vi "SSL Detection Frame Simple Estimator Kalman.vi"(7 "Enable":bool, 10 "Field Size":T1, 11 "Detection Frame In":T2 {"robots_blue"."height" format="%+4.3f"; "robots_blue"."pixel_y" format="%+4.3f"; "robots_blue"."pixel_x" format="%+4.3f"; "robots_blue"."orientation" format="%+4.3f"; "robots_blue"."y" format="%+4.3f"; "robots_blue"."confidence" format="%4.3f"; "robots_blue"."x" format="%+4.3f"; "robots_yellow"."height" format="%+4.3f"; "robots_yellow"."pixel_y" format="%+4.3f"; "robots_yellow"."pixel_x" format="%+4.3f"; "robots_yellow"."orientation" format="%+4.3f"; "robots_yellow"."y" format="%+4.3f"; "robots_yellow"."confidence" format="%4.3f"; "robots_yellow"."x" format="%+4.3f"}) -> (2 "Field Size Out":T1, 3 "Detection Frame Out":T2 {"robots_blue"."height" format="%+4.3f"; "robots_blue"."pixel_y" format="%+4.3f"; "robots_blue"."pixel_x" format="%+4.3f"; "robots_blue"."orientation" format="%+4.3f"; "robots_blue"."y" format="%+4.3f"; "robots_blue"."confidence" format="%4.3f"; "robots_blue"."x" format="%+4.3f"; "robots_yellow"."height" format="%+4.3f"; "robots_yellow"."pixel_y" format="%+4.3f"; "robots_yellow"."pixel_x" format="%+4.3f"; "robots_yellow"."orientation" format="%+4.3f"; "robots_yellow"."y" format="%+4.3f"; "robots_yellow"."confidence" format="%4.3f"; "robots_yellow"."x" format="%+4.3f"})   [LabVIEW 2016]
uses:
  SSL Detection Frame.ctl
  SSL Detection Robot.ctl
  SSL Detection Ball.ctl
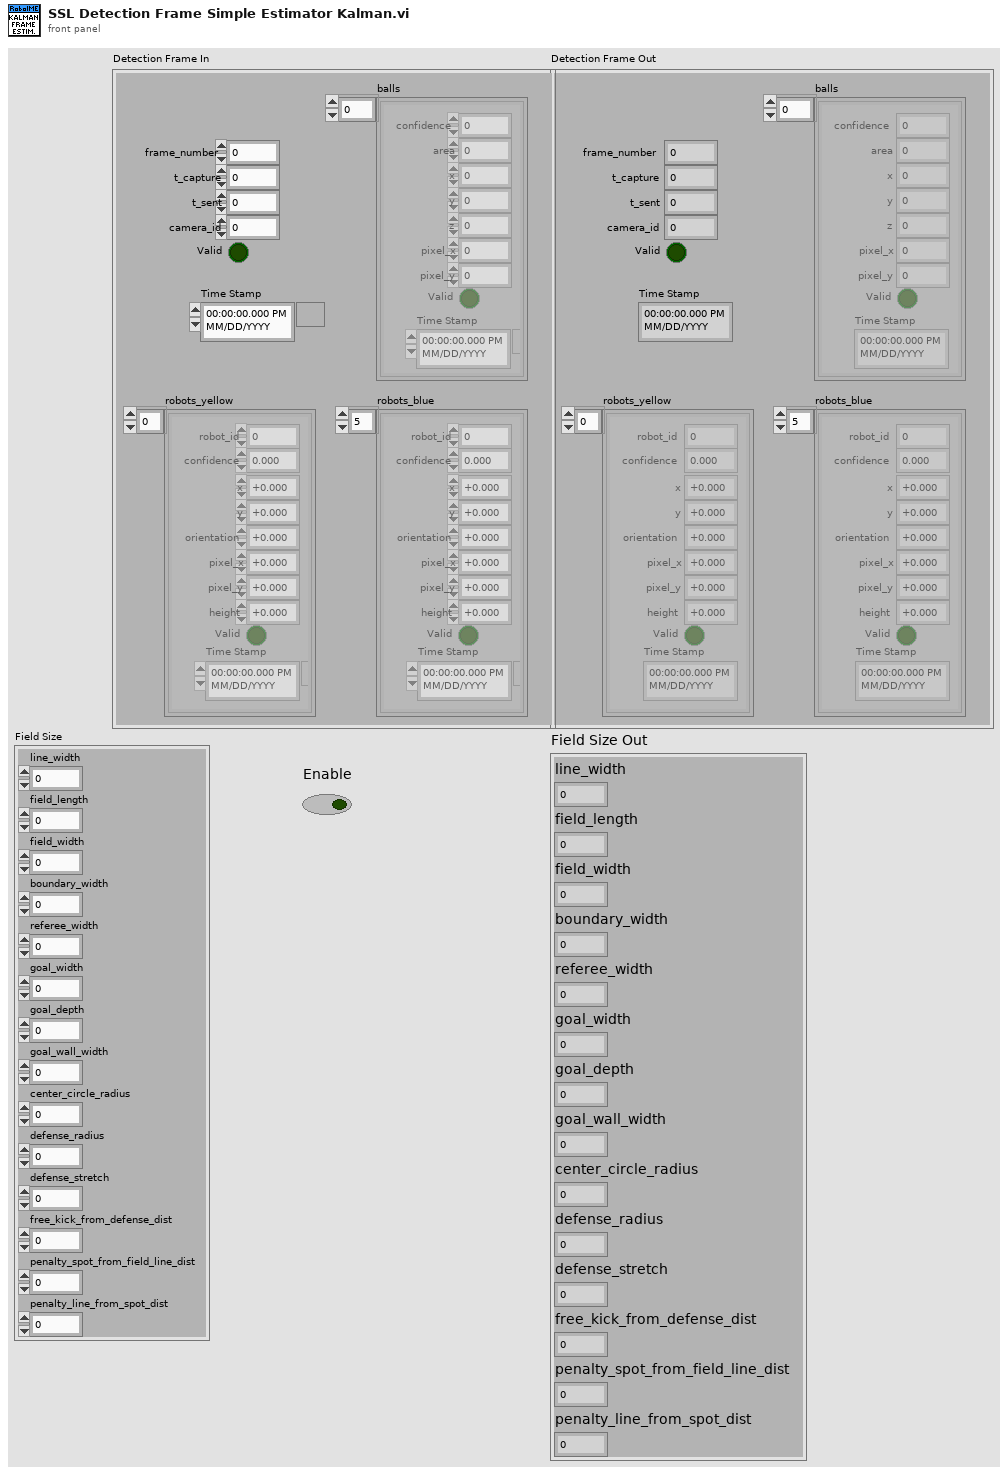
[diagram p1: front panel]
types:
  T1 = cluster{"line_width":u32, "field_length":u32, "field_width":u32, "boundary_width":u32, "referee_width":u32, "goal_width":u32, "goal_depth":u32, "goal_wall_width":u32, "center_circle_radius":u32, "defense_radius":u32, "defense_stretch":u32, "free_kick_from_defense_dist":u32, "penalty_spot_from_field_line_dist":u32, "penalty_line_from_spot_dist":u32}
  T2 = typedef "SSL Detection Frame.ctl" = cluster{"frame_number":u32, "t_capture":dbl, "t_sent":dbl, "camera_id":u32, "robots_yellow":T3[], "robots_blue":T3[], "balls":T4[], "Valid":bool, "Time Stamp":timestamp}
  T3 = typedef "SSL Detection Robot.ctl" = cluster{"x":sgl, "robot_id":u32, "confidence":sgl, "y":sgl, "orientation":sgl, "pixel_x":sgl, "pixel_y":sgl, "height":sgl, "Valid":bool, "Time Stamp":timestamp}
  T4 = typedef "SSL Detection Ball.ctl" = cluster{"x":sgl, "area":u32, "confidence":sgl, "y":sgl, "z":sgl, "pixel_x":sgl, "pixel_y":sgl, "Valid":bool, "Time Stamp":timestamp}
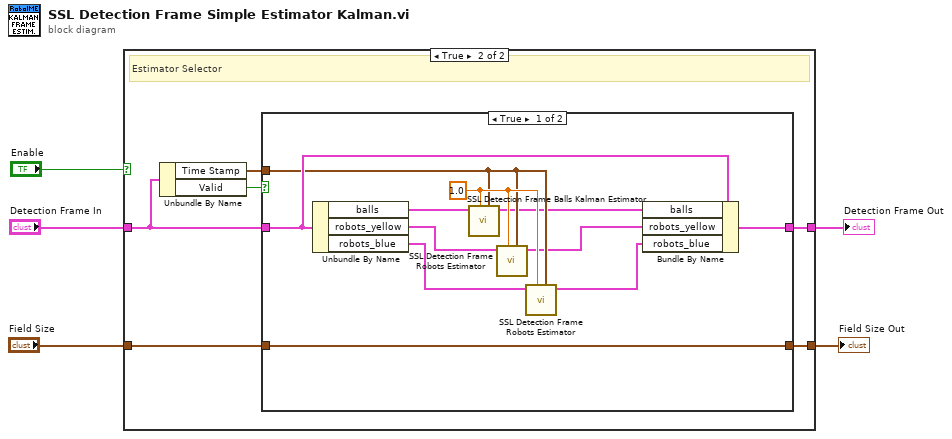
[diagram p0: block diagram]
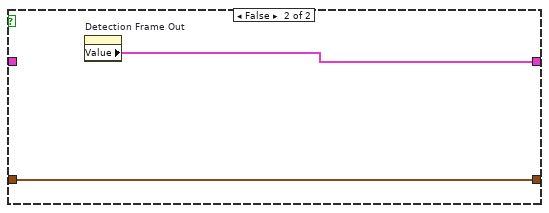
[diagram p3: hidden frame]
diagram:
  n1 = case shown="True" "Enable" {
    tunnel: [w7 w13] -> w5
    tunnel: "Detection Frame In" -> [w7 w10]
    tunnel: "Field Size" -> [w6 w12]
    tunnel: [w6 w11] -> w2
    frame False {
    }
    frame True {
      # "Estimator Selector"
      n2 = Unbundle By Name(w10) -> ("Time Stamp"=w8:timestamp, "Valid"=w9:bool)
      n3 = case shown="True" w9 {
        tunnel: w10 -> [w24 _]
        tunnel: [w23 w26] -> w13
        tunnel: w8 -> [w18 _]
        tunnel: w12 -> [w15 w25]
        tunnel: [w15 w25] -> w11
        frame True {
          w19 = 1.0 ("Life Time")
          n4 = Unbundle By Name(w24) -> ("balls"=w21:T4[], "robots_yellow"=w22:T3[], "robots_blue"=w20:T3[])
          n5 = call "SSL Detection Frame Balls Kalman Estimator.vi"("Time Stamp 2"=w18, "Life Time 2"=w19, "balls"=w21) -> ("Array 2"=w14:T4[])  [unwired: 8 in]
          n6 = call "SSL Detection Frame Robots Estimator.vi"("Time Stamp"=w18, "Life Time"=w19, "Robots"=w22) -> ("Est. Robots"=w17:T3[])  [unwired: 8 in]
          n7 = call "SSL Detection Frame Robots Estimator.vi"("Time Stamp"=w18, "Life Time"=w19, "Robots"=w20) -> ("Est. Robots"=w16:T3[])  [unwired: 8 in]
          n8 = Bundle By Name(cluster=w24, "balls"=w14, "robots_yellow"=w17, "robots_blue"=w16) -> (w23:T2)
        }
        frame False {
          n9 = property on="Detection Frame Out" class="Clust (strict)"() -> ("Value"=w26:T2)  [unwired: 2 in, 2 out]
        }
      }
    }
  }
  "Detection Frame Out" <- w5
  "Field Size Out" <- w2
